vi "Write DAQmx Task.vi"(8 "error in (no error)":errorcluster, 10 "DAQmx Task":refnum<k21>, 11 "DAQmx Actor in":refnum<class "DAQmx Actor.lvclass">) -> (0 "error out":errorcluster, 3 "DAQmx Actor out":refnum<class "DAQmx Actor.lvclass">)   [LabVIEW 2024, in "DAQmx Actor.lvlib" / "DAQmx Actor.lvclass"]
uses:
  DAQmx Actor.lvclass
  DAQmx Actor.lvclass/DAQmx Actor.ctl
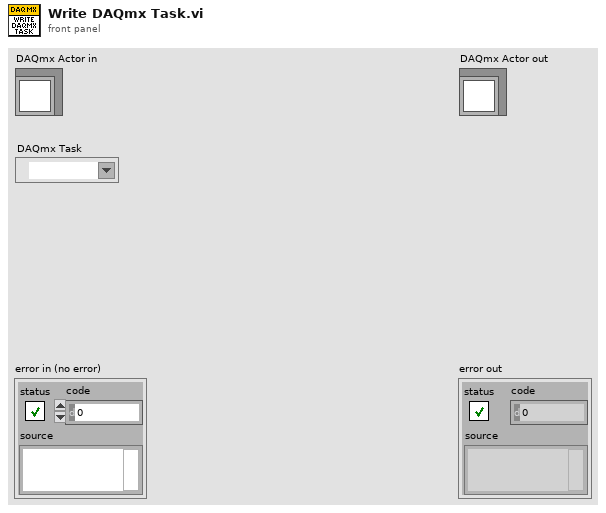
[diagram p1: front panel]
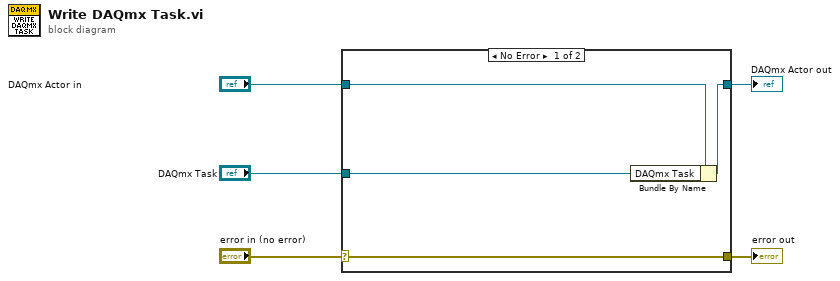
[diagram p0: block diagram]
diagram:
  n1 = case shown="No Error" "error in (no error)" {
    selector: "error in (no error)" -> [w9 w10]
    tunnel: [w9 w10] -> w4
    tunnel: [w7 w11] -> w2
    tunnel: "DAQmx Actor in" -> [w8 w11]
    tunnel: "DAQmx Task" -> [w6 _]
    frame No Error {
      n2 = Bundle By Name(cluster=w8, "DAQmx Task"=w6) -> (w7:refnum<class "DAQmx Actor.lvclass">)
    }
    frame Error {
    }
  }
  "error out" <- w4
  "DAQmx Actor out" <- w2
